vi "Get Plot at Mouse Click [AAC].vi"(8 "error in (no error)":errorcluster, 10 "Mouse Click Coordinates":T1, 11 "XYGraph Ref":T2) -> (0 "error out":errorcluster, 1 "Click is in Legend?":bool, 2 "Plot at Coordinates":i32, 3 "XYGraph Ref":T2, 4 "Plot Name":string, 5 "Graph Name":string, 6 "Found?":bool)   [LabVIEW 2019]
uses:
  XY Graph/XY Graph Refnum.ctl
  <vilib>/Utility/miscctls.llb/LVPoint32TypeDef.ctl
  <vilib>/Utility/error.llb/Error Cluster From Error Code.vi
  <vilib>/ErrorRing/Error Ring.xnode
  XY Graph/XY Graph Add-Ons.lvlib
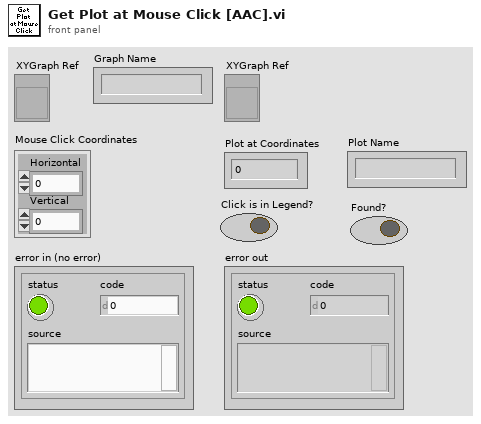
[diagram p1: front panel]
types:
  T1 = typedef "LVPoint32TypeDef.ctl" = cluster{"Horizontal":i32, "Vertical":i32}
  T2 = typedef "XY Graph Add-Ons.lvlib/XY Graph Refnum.ctl" = refnum<vi>
  T3 = typedef "LVPositionTypeDef.ctl" = cluster{"Left":i32, "Top":i32}
  T4 = typedef "LVBoundsTypeDef.ctl" = cluster{"Width":u32, "Height":u32}
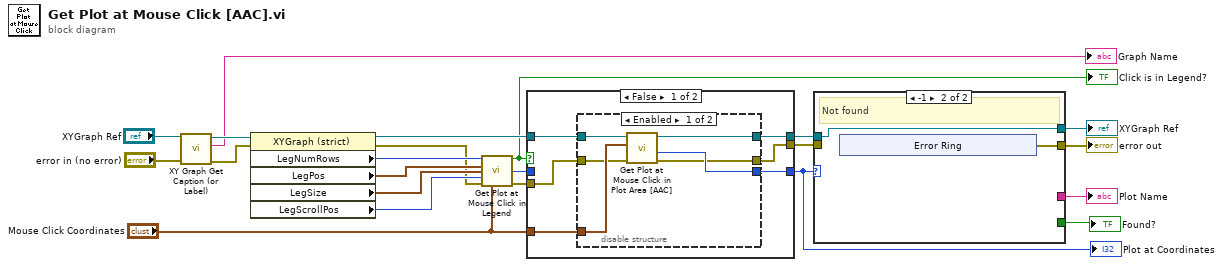
[diagram p0: block diagram]
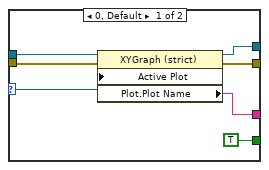
[diagram p2: hidden frame]
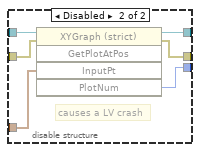
[diagram p3: hidden frame]
diagram:
  n1 = call "XY Graph Get Caption (or Label).vi"("error in (no error)"="error in (no error)", "XYGraph in"="XYGraph Ref") -> ("error out"=w3:errorcluster, "Caption (or Label) Text"=→"Graph Name":string, "XYGraph out"=w2:T2)  [unwired: 7 in]
  n2 = property class="XYGraph (strict)"(reference=w2, error in=w3) -> (reference out=w20:T2, error out=w13:errorcluster, "LegNumRows"=w21:u32, "LegPos"=w18:T3, "LegSize"=w17:T4, "LegScrollPos"=w16:u32)
  n3 = call "Get Plot at Mouse Click in Legend.vi"("LegNumRows"=w21, "Legend:Position"=w18, "Legend:Size"=w17, "LegScrollPos"=w16, "Error In"=w13, "Mouse Click Coordinates"="Mouse Click Coordinates") -> ("Click is in Legend?"=w19:bool, "Plot Index"=w14:i32, "Error Out"=w12:errorcluster)  [unwired: 7 in]
  "Click is in Legend?" <- w19
  n4 = case shown="False" w19 {
    tunnel: w20 -> [w25 w43]
    tunnel: [w28 w43] -> w22
    tunnel: w14 -> [_ w42]
    tunnel: [w27 w42] -> w8
    tunnel: "Mouse Click Coordinates" -> [w26 _]
    tunnel: w12 -> [w24 w41]
    tunnel: [w23 w41] -> w10
    frame False {
      n5 = disable-structure shown="Enabled" {
        disable-tunnel: [w34 w39] -> w28
        disable-tunnel: [w33 w35] -> w27
        disable-tunnel: w26 -> [w32 w37]
        disable-tunnel: w25 -> [w31 w40]
        disable-tunnel: w24 -> [w30 w38]
        disable-tunnel: [w29 w36] -> w23
        frame Enabled {
          n6 = call "Get Plot at Mouse Click in Plot Area [AAC].vi"("error in (no error)"=w30, "Mouse Click Coordinates (defaut: last plot)"=w32, "XYGraph Ref"=w31) -> ("error out"=w29:errorcluster, "Plot Index"=w33:i32, "XYGraph Ref"=w34:T2)  [unwired: 6 in]
        }
        frame Disabled {
          # "causes a LV crash"
          n7 = invoke class="XYGraph (strict)" method="GetPlotAtPos"(reference=w40, error in=w38, "InputPt"=w37) -> (reference out=w39:T2, error out=w36:errorcluster, "PlotNum"=w35:i32)  [unwired: 2 in, 2 out]
        }
      }
    }
    frame True {
      # "In the Legend Region"
    }
  }
  "Plot at Coordinates" <- w8
  n8 = case shown="-1" w8 {
    selector: w8 -> [w46 _]
    tunnel: w22 -> [w50 w52]
    tunnel: [w49 w52] -> w11
    tunnel: w10 -> [w48 _]
    tunnel: [w47 w51] -> w9
    tunnel: [w45 _] -> w7
    tunnel: [TRUE ("Found?") _] -> w6
    frame 0, Default {
      n9 = property class="XYGraph (strict)"(reference=w50, error in=w48, "Active Plot"=w46) -> (reference out=w49:T2, error out=w47:errorcluster, "Plot.Plot Name"=w45:string)
    }
    frame -1 {
      # "Not found"
      n10 = xnode "Error Ring"() -> ("error out"=w51:errorcluster)
    }
  }
  "error out" <- w9
  "XYGraph Ref" <- w11
  "Plot Name" <- w7
  "Found?" <- w6
